vi "i2clib_write.vi"(8 "error in (no error)":errorcluster, 9 "send_data":u8[](array[numeric]), 10 "dev_addr":u8, 11 "I2C Reference":i32) -> (0 "error out":errorcluster, 3 "I2C Reference Out":i32)   [LabVIEW 2017]
uses:
  <vilib>/Utility/error.llb/Error Cluster From Error Code.vi
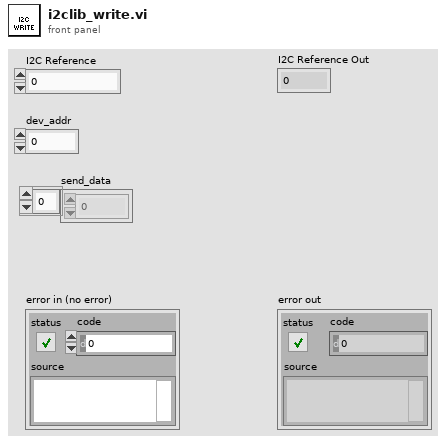
[diagram p1: front panel]
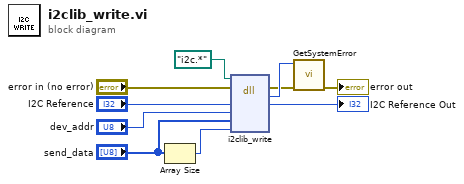
[diagram p0: block diagram]
diagram:
  n1 = Array Size(array="send_data") -> (size(s)=w7:i32)
  n2 = dll-call lib="?" fn="i2clib_write"(path in=path "i2c.*", error in="error in (no error)", "handle"="I2C Reference", "dev_addr"="dev_addr", "send_buf"="send_data", "send_size"=w7) -> (error out=w2:errorcluster, "return type"=w3:i32, "handle"=→"I2C Reference Out":i32)  [unwired: 4 in, 1 out]
  n3 = call <vilib>:"GetSystemError.vi"("error in (no error)"=w2, "Retval"=w3) -> ("error out"=→"error out":errorcluster)  [unwired: 9 in]
